vi "constructDistance.vi"(2 "distance_front":cluster{"left":dbl, "middle":dbl, "right":dbl}, 3 "distance_back":cluster{"left":dbl, "middle":dbl, "right":dbl}) -> (0 "Ultrasonics":T1, 1 "Lasers":T1)   [LabVIEW 2016]
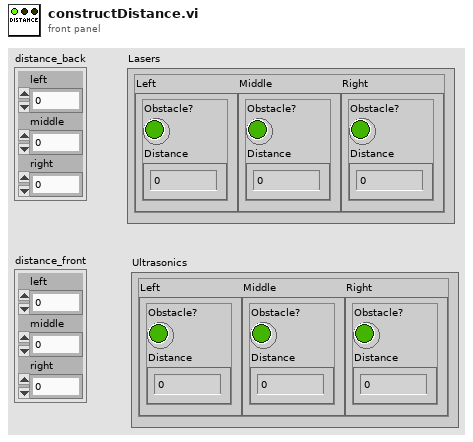
[diagram p1: front panel]
types:
  T1 = cluster{"Left":cluster{"Obstacle?":bool, "Distance":dbl}, "Middle":cluster{"Obstacle?":bool, "Distance":dbl}, "Right":cluster{"Obstacle?":bool, "Distance":dbl}}
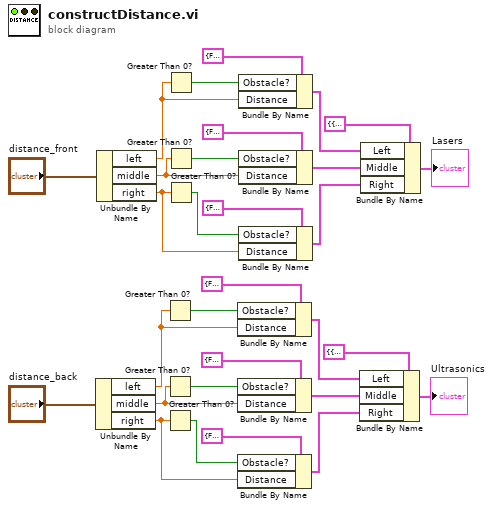
[diagram p0: block diagram]
diagram:
  n1 = Unbundle By Name("distance_back") -> ("left"=w15:dbl, "middle"=w13:dbl, "right"=w12:dbl)
  n2 = Unbundle By Name("distance_front") -> ("left"=w26:dbl, "middle"=w22:dbl, "right"=w20:dbl)
  n3 = Greater Than 0?(x=w15) -> (x > 0?=w16:bool)
  n4 = Greater Than 0?(x=w13) -> (x > 0?=w14:bool)
  n5 = Greater Than 0?(x=w12) -> (x > 0?=w11:bool)
  n6 = Greater Than 0?(x=w26) -> (x > 0?=w27:bool)
  n7 = Greater Than 0?(x=w22) -> (x > 0?=w23:bool)
  n8 = Greater Than 0?(x=w20) -> (x > 0?=w21:bool)
  n9 = Bundle By Name(cluster=cluster{"Obstacle?":bool, "Distance":dbl} {"Obstacle?"=FALSE, "Distance"=0.0}, "Obstacle?"=w16, "Distance"=w15) -> (w5:cluster{"Obstacle?":bool, "Distance":dbl})
  n10 = Bundle By Name(cluster=cluster{"Obstacle?":bool, "Distance":dbl} {"Obstacle?"=FALSE, "Distance"=0.0}, "Obstacle?"=w14, "Distance"=w13) -> (w4:cluster{"Obstacle?":bool, "Distance":dbl})
  n11 = Bundle By Name(cluster=cluster{"Obstacle?":bool, "Distance":dbl} {"Obstacle?"=FALSE, "Distance"=0.0}, "Obstacle?"=w11, "Distance"=w12) -> (w3:cluster{"Obstacle?":bool, "Distance":dbl})
  n12 = Bundle By Name(cluster=cluster{"Obstacle?":bool, "Distance":dbl} {"Obstacle?"=FALSE, "Distance"=0.0}, "Obstacle?"=w27, "Distance"=w26) -> (w8:cluster{"Obstacle?":bool, "Distance":dbl})
  n13 = Bundle By Name(cluster=cluster{"Obstacle?":bool, "Distance":dbl} {"Obstacle?"=FALSE, "Distance"=0.0}, "Obstacle?"=w23, "Distance"=w22) -> (w7:cluster{"Obstacle?":bool, "Distance":dbl})
  n14 = Bundle By Name(cluster=cluster{"Obstacle?":bool, "Distance":dbl} {"Obstacle?"=FALSE, "Distance"=0.0}, "Obstacle?"=w21, "Distance"=w20) -> (w6:cluster{"Obstacle?":bool, "Distance":dbl})
  n15 = Bundle By Name(cluster=T1 {"Left"={"Obstacle?"=FALSE, "Distance"=0.0}, "Middle"={"Obstacle?"=FALSE, "Distance"=0.0}, "Right"={"Obstacle?"=FALSE, "Distance"=0.0}}, "Left"=w5, "Middle"=w4, "Right"=w3) -> (→"Ultrasonics":T1)
  n16 = Bundle By Name(cluster=T1 {"Left"={"Obstacle?"=FALSE, "Distance"=0.0}, "Middle"={"Obstacle?"=FALSE, "Distance"=0.0}, "Right"={"Obstacle?"=FALSE, "Distance"=0.0}}, "Left"=w8, "Middle"=w7, "Right"=w6) -> (→"Lasers":T1)
